vi "create SubFolder.vi"(8 "Fehler (Eingang)":errorcluster, 10 "Ordner":string="SysLog", 11 "Pfad":string="D:\\IAG_DATA\\Log\\") -> (0 "Fehler (Ausgang)":errorcluster, 2 "SubOrdner":string, 3 "Ordnernamen":string[](array[string]))   [LabVIEW 2020, in "allgemeine Sub-VIs.lvlib"]
doc: "Erzeugt einen SubOrdner, wenn er noch nicht existiert.\nPfad: D:\\IAG_DATA\\\nOrdner: SysLog\nFehler (Ausgang)\n\nriw 21.09.2018"
uses:
  allgemeine Sub-VIs.lvlib
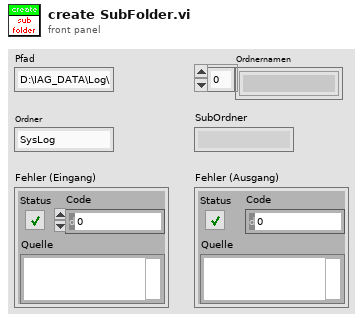
[diagram p1: front panel]
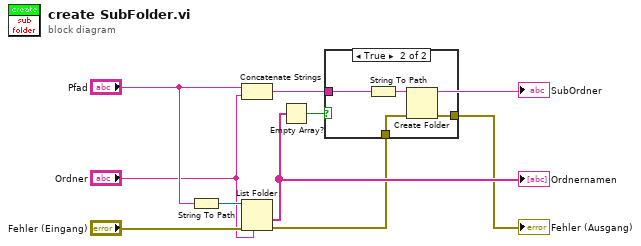
[diagram p0: block diagram]
diagram:
  n1 = String To Path(string="Pfad") -> (path=w9:path)
  n2 = Concatenate Strings("Pfad", "Ordner") -> (w7:string)
  "SubOrdner" <- w7
  n3 = List Folder(path=w9, pattern="Ordner", error in="Fehler (Eingang)") -> (folder names=w6:string[], error out=w5:errorcluster)  [unwired: 1 in, 2 out]
  "Ordnernamen" <- w6
  n4 = Empty Array?(array=w6) -> (empty?=w8:bool)
  n5 = case shown="True" w8 {
    tunnel: w7 -> [_ w13]
    tunnel: w5 -> [_ w11]
    tunnel: [_ w10] -> w4
    frame False {
    }
    frame True {
      n6 = String To Path(string=w13) -> (path=w12:path)
      n7 = Create Folder(path (use dialog)=w12, error in=w11) -> (error out=w10:errorcluster)  [unwired: 1 in, 2 out]
    }
  }
  "Fehler (Ausgang)" <- w4
